vi "ControlsToCluster.vi"(10 "Path (px)":cluster{dbl, dbl}[](array[cluster]), 11 "Path (in)":cluster{dbl, dbl}[](array[cluster])) -> (3 "Path File Data":T1={"RobotNeeded"={"Path"=[], "MaxVel"=0.0, "MaxAccel"=0.0, "Backwards?"=FALSE, "PointSpacing"=0.0, "LookaheadDist"=0.0, "Speed/Curve"=1.8, "SlowDistanceAtEnd"=12.0, "SlowSpeed"=15.0, "MaxDeAccel"=0.0}, "Meta"={"Path (px)"=[], "RobotWidth"=0.0, "RobotLength"=0.0, "CenterOfRotYOffset"=0.0, "Roundedness"=0.0, "StartingPositionPreset"=0}} {"RobotNeeded"."SlowSpeed" format="%#_13g"; "RobotNeeded"."SlowDistanceAtEnd" format="%#_13g"; "RobotNeeded"."Speed/Curve" format="%#_13g"})   [LabVIEW 2018]
uses:
  Dawgma Programming Library/Controls/PurePursuit/PathFileData.ctl
  Dawgma Programming Library/Controls/PurePursuit/RobotNeededPathData.ctl
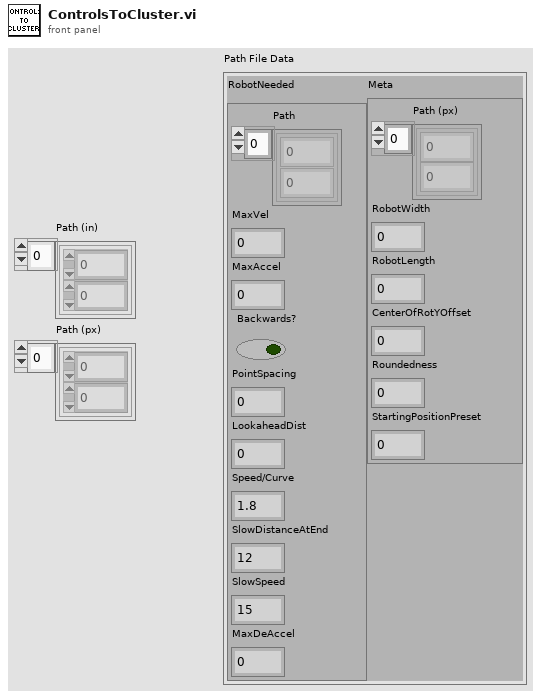
[diagram p1: front panel]
types:
  T1 = typedef "PathFileData.ctl" = cluster{"RobotNeeded":T2, "Meta":cluster{"Path (px)":cluster{i32, i32}[], "RobotWidth":dbl, "RobotLength":dbl, "CenterOfRotYOffset":dbl, "Roundedness":dbl, "StartingPositionPreset":u32}}
  T2 = typedef "RobotNeededPathData.ctl" = cluster{"Path":cluster{dbl, dbl}[], "MaxVel":dbl, "MaxAccel":dbl, "Backwards?":bool, "PointSpacing":dbl, "LookaheadDist":dbl, "Speed/Curve":dbl, "SlowDistanceAtEnd":dbl, "SlowSpeed":dbl, "MaxDeAccel":dbl}
  T3 = cluster{"Path (px)":cluster{i32, i32}[], "RobotWidth":dbl, "RobotLength":dbl, "CenterOfRotYOffset":dbl, "Roundedness":dbl, "StartingPositionPreset":u32, "PathName":string}
  T4 = cluster{"Path (px)":cluster{i32, i32}[], "RobotWidth":dbl, "RobotLength":dbl, "CenterOfRotYOffset":dbl, "Roundedness":dbl, "StartingPositionPreset":u32}
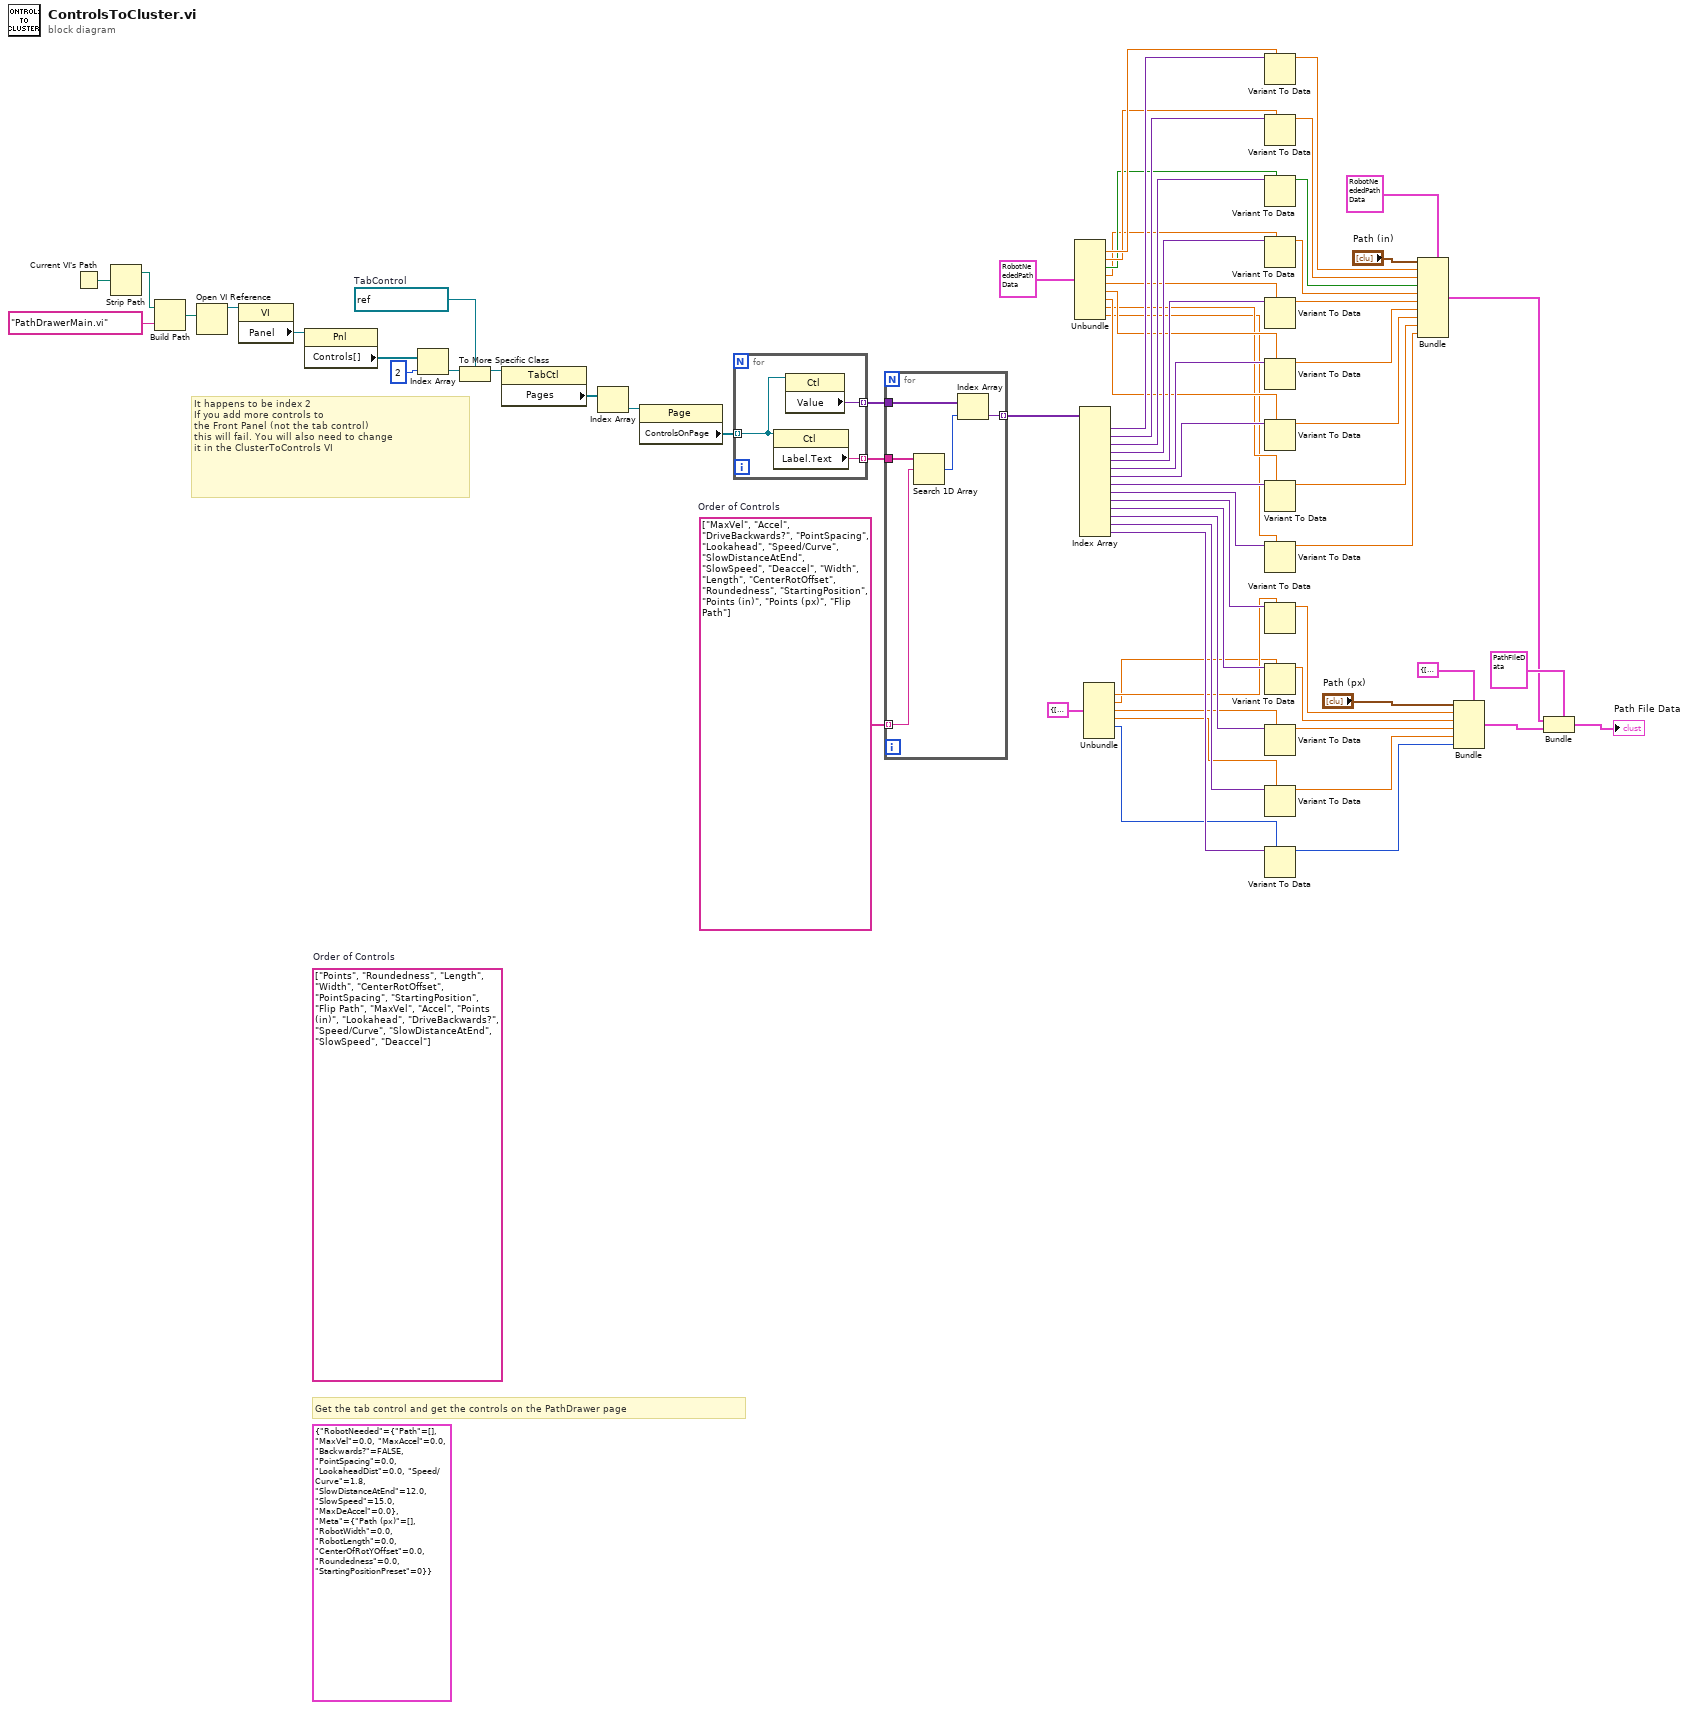
[diagram p0: block diagram]
diagram:
  w43 = string[] ["MaxVel", "Accel", "DriveBackwards?", "PointSpacing", "Lookahead", "Speed/Curve", "SlowDistanceAtEnd", "SlowSpeed", "Deaccel", "Width", "Length", "CenterRotOffset", "Roundedness", "StartingPosition", "Points (in)", "Points (px)", "Flip Path"]  # Order of Controls
  (unwired) string[] ["Points", "Roundedness", "Length", "Width", "CenterRotOffset", "PointSpacing", "StartingPosition", "Flip Path", "MaxVel", "Accel", "Points (in)", "Lookahead", "DriveBackwards?", "Speed/Curve", "SlowDistanceAtEnd", "SlowSpeed", "Deaccel"]  # Order of Controls
  w69 = refnum<vi> refnum  # TabControl
  (unwired) T1 {"RobotNeeded"={"Path"=[], "MaxVel"=0.0, "MaxAccel"=0.0, "Backwards?"=FALSE, "PointSpacing"=0.0, "LookaheadDist"=0.0, "Speed/Curve"=1.8, "SlowDistanceAtEnd"=12.0, "SlowSpeed"=15.0, "MaxDeAccel"=0.0}, "Meta"={"Path (px)"=[], "RobotWidth"=0.0, "RobotLength"=0.0, "CenterOfRotYOffset"=0.0, "Roundedness"=0.0, "StartingPositionPreset"=0}} ("Data")
  # "It happens to be index 2\nIf you add more controls to\nthe Front Panel (not the tab control)\nthis will fail. You will also need to change\nit in the ClusterToControls VI"
  # "Get the tab control and get the controls on the PathDrawer page"
  n1 = Current VI's Path() -> (path=w6:path)
  n2 = Strip Path(path=w6) -> (stripped path=w5:path)  [unwired: 1 out]
  n3 = Build Path(base path=w5, name or relative path="PathDrawerMain.vi") -> (appended path=w3:path)
  n4 = Open VI Reference(vi path=w3) -> (vi reference=w2:refnum<vi>)  [unwired: 5 in, 1 out]
  n5 = property class="VI"(reference=w2) -> ("Panel"=w7:refnum<vi>)  [unwired: 1 in, 2 out]
  n6 = property class="Pnl"(reference=w7) -> ("Controls[]"=w1:refnum<vi>[])  [unwired: 1 in, 2 out]
  n7 = Index Array(array=w1, index=2) -> (element=w68:refnum<vi>)
  n8 = To More Specific Class(target class=w69, reference=w68) -> (specific class reference=w67:refnum<vi>)  [unwired: 1 in, 1 out]
  n9 = property class="TabCtl"(reference=w67) -> ("Pages"=w66:refnum<vi>[])  [unwired: 1 in, 2 out]
  n10 = Index Array(array=w66) -> (element=w65:refnum<vi>)  [unwired: 1 in]
  n11 = property class="Page"(reference=w65) -> ("ControlsOnPage"=w64:refnum<vi>[])  [unwired: 1 in, 2 out]
  n12 = for {
    tunnel: w64 -> [w72] mode=indexing
    tunnel: [w73] -> w44 mode=indexing
    tunnel: [w71] -> w45 mode=indexing
    n13 = property class="Ctl"(reference=w72) -> ("Label.Text"=w73:string)  [unwired: 1 in, 2 out]
    n14 = property class="Ctl"(reference=w72) -> ("Value"=w71:variant)  [unwired: 1 in, 2 out]
  }
  n15 = for {
    tunnel: [w74] -> w46 mode=indexing
    tunnel: w45 -> [w76]
    tunnel: w44 -> [w78]
    tunnel: w43 -> [w77] mode=indexing
    n16 = Search 1D Array(1D array=w78, element=w77) -> (index of element=w75:i32)  [unwired: 1 in]
    n17 = Index Array(array=w76, index=w75) -> (element=w74:variant)
  }
  n18 = Unbundle(T2 {"Path"=[], "MaxVel"=0.0, "MaxAccel"=0.0, "Backwards?"=FALSE, "PointSpacing"=0.0, "LookaheadDist"=0.0, "Speed/Curve"=1.8, "SlowDistanceAtEnd"=12.0, "SlowSpeed"=15.0, "MaxDeAccel"=0.0} ("RobotNeededPathData")) -> ("MaxVel"=w42:dbl, "MaxAccel"=w40:dbl, "Backwards?"=w37:bool, "PointSpacing"=w36:dbl, "LookaheadDist"=w33:dbl, "Speed/Curve"=w32:dbl, "SlowDistanceAtEnd"=w30:dbl, "SlowSpeed"=w27:dbl, "MaxDeAccel"=w26:dbl)  [unwired: 1 out]
  n19 = Index Array(array=w46) -> (element #1=w63:variant, element #2=w62:variant, element #3=w61:variant, element #4=w60:variant, element #5=w59:variant, element #6=w58:variant, element #7=w57:variant, element #8=w56:variant, element #9=w55:variant, element #10=w54:variant, element #11=w53:variant, element #12=w52:variant, element #13=w51:variant, element #14=w47:variant)  [unwired: 14 in]
  n20 = Unbundle(T3 {"Path (px)"=[], "RobotWidth"=0.0, "RobotLength"=0.0, "CenterOfRotYOffset"=0.0, "Roundedness"=0.0, "StartingPositionPreset"=0, "PathName"=""} ("Meta")) -> ("RobotWidth"=w19:dbl, "RobotLength"=w16:dbl, "CenterOfRotYOffset"=w15:dbl, "Roundedness"=w14:dbl, "StartingPositionPreset"=w13:u32)  [unwired: 2 out]
  n21 = Variant To Data(type=w42, Variant=w63) -> (data=w41:dbl)  [unwired: 1 in, 1 out]
  n22 = Variant To Data(type=w40, Variant=w62) -> (data=w39:dbl)  [unwired: 1 in, 1 out]
  n23 = Variant To Data(type=w37, Variant=w61) -> (data=w38:bool)  [unwired: 1 in, 1 out]
  n24 = Variant To Data(type=w36, Variant=w60) -> (data=w35:dbl)  [unwired: 1 in, 1 out]
  n25 = Variant To Data(type=w33, Variant=w59) -> (data=w34:dbl)  [unwired: 1 in, 1 out]
  n26 = Variant To Data(type=w32, Variant=w58) -> (data=w31:dbl)  [unwired: 1 in, 1 out]
  n27 = Variant To Data(type=w30, Variant=w57) -> (data=w29:dbl)  [unwired: 1 in, 1 out]
  n28 = Variant To Data(type=w27, Variant=w56) -> (data=w28:dbl)  [unwired: 1 in, 1 out]
  n29 = Variant To Data(type=w26, Variant=w55) -> (data=w25:dbl)  [unwired: 1 in, 1 out]
  n30 = Variant To Data(type=w19, Variant=w54) -> (data=w18:dbl)  [unwired: 1 in, 1 out]
  n31 = Variant To Data(type=w16, Variant=w53) -> (data=w17:dbl)  [unwired: 1 in, 1 out]
  n32 = Variant To Data(type=w15, Variant=w52) -> (data=w10:dbl)  [unwired: 1 in, 1 out]
  n33 = Variant To Data(type=w14, Variant=w51) -> (data=w11:dbl)  [unwired: 1 in, 1 out]
  n34 = Variant To Data(type=w13, Variant=w47) -> (data=w12:u32)  [unwired: 1 in, 1 out]
  n35 = Bundle(cluster=T2 {"Path"=[], "MaxVel"=0.0, "MaxAccel"=0.0, "Backwards?"=FALSE, "PointSpacing"=0.0, "LookaheadDist"=0.0, "Speed/Curve"=1.8, "SlowDistanceAtEnd"=12.0, "SlowSpeed"=15.0, "MaxDeAccel"=0.0} ("RobotNeededPathData"), "Path"="Path (in)", "MaxVel"=w41, "MaxAccel"=w39, "Backwards?"=w38, "PointSpacing"=w35, "LookaheadDist"=w34, "Speed/Curve"=w31, "SlowDistanceAtEnd"=w29, "SlowSpeed"=w28, "MaxDeAccel"=w25) -> (w9:T2)
  n36 = Bundle(cluster=T4 {"Path (px)"=[], "RobotWidth"=0.0, "RobotLength"=0.0, "CenterOfRotYOffset"=0.0, "Roundedness"=0.0, "StartingPositionPreset"=0} ("Meta"), "Path (px)"="Path (px)", "RobotWidth"=w18, "RobotLength"=w17, "CenterOfRotYOffset"=w10, "Roundedness"=w11, "StartingPositionPreset"=w12) -> (w23:T4)
  n37 = Bundle(cluster=T1 {"RobotNeeded"={"Path"=[], "MaxVel"=0.0, "MaxAccel"=0.0, "Backwards?"=FALSE, "PointSpacing"=0.0, "LookaheadDist"=0.0, "Speed/Curve"=1.8, "SlowDistanceAtEnd"=12.0, "SlowSpeed"=15.0, "MaxDeAccel"=0.0}, "Meta"={"Path (px)"=[], "RobotWidth"=0.0, "RobotLength"=0.0, "CenterOfRotYOffset"=0.0, "Roundedness"=0.0, "StartingPositionPreset"=0}} ("Data"), "RobotNeeded"=w9, "Meta"=w23) -> (→"Path File Data":T1)
